vi "Get Magnet Field.vi"(6 "Axis":T1, 8 "error in (no error)":errorcluster, 11 "instrument.PPMS2 in":refnum<class "instrument.PPMS2.lvclass">) -> (0 "error out":errorcluster, 1 "Status":variant, 2 "B Field (T)":dbl, 3 "instrument.PPMS2 out":refnum<class "instrument.PPMS2.lvclass">, 4 "Finished?":bool)   [LabVIEW 2016, in "instrument.PPMS2.lvclass"]
uses:
  instrument.PPMS2.lvclass
  <userlib>/LevyLab/Levylab Instruments/Instrument Types/Cryostat/Typedefs/Magnet Axis--Enum.ctl
  Typedefs/PPMS2.Magnet Status--cluster.ctl
  Typedefs/PPMS2.Commands-enum.ctl
  <userlib>/LevyLab/Levylab Instruments/Instrument Types/Cryostat/Instrument.Cryostat.lvclass
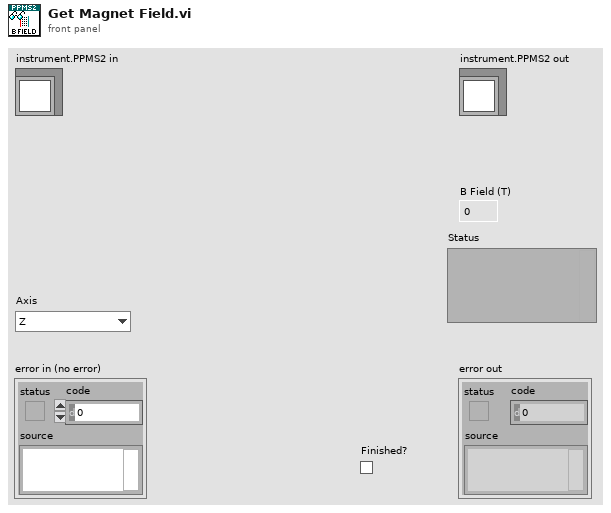
[diagram p1: front panel]
types:
  T1 = typedef "Instrument.Cryostat.lvclass/Magnet Axis--Enum.ctl" = enum16{"Z", "X", "Y"}
  T2 = typedef "instrument.PPMS2.lvclass/PPMS2.Commands-enum.ctl" = enum16{"Get Magnet Field", "Get Helium Level", "Get Temperature", "Get Angle", "Set Magnet Field", "Set Temperature", "Set Angle", "getAll"}
  T3 = typedef "instrument.PPMS2.lvclass/PPMS2.Magnet Status--cluster.ctl" = cluster{"Field (Oe)":dbl, "Magnet Status":string}
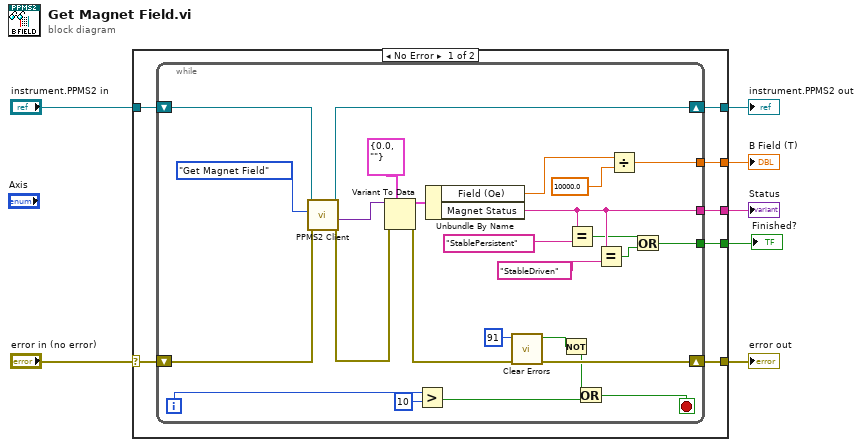
[diagram p0: block diagram]
diagram:
  n1 = case shown="No Error" "error in (no error)" {
    selector: "error in (no error)" -> [w9 w41]
    tunnel: [w10 w41] -> w7
    tunnel: [w14 w42] -> w6
    tunnel: "instrument.PPMS2 in" -> [w13 w42]
    tunnel: [w12 _] -> w4
    tunnel: [w11 _] -> w3
    tunnel: [w8 _] -> w1
    frame No Error {
      n2 = while {
        tunnel: [w25] -> w12
        tunnel: [w34] -> w11
        shift-right: [w29] -> w10
        shift-left: w9 -> [w39]
        shift-right: [w38] -> w14
        shift-left: w13 -> [w37]
        tunnel: [w21] -> w8
        i -> [w16]
        stop <- w15 stop-if-true
        n3 = call "PPMS2 Client.vi"("error in (no error)"=w39, "Command"=PPMS2.Commands-enum."Get Magnet Field" ("Enum"), "instrument.PPMS2 in"=w37) -> ("error out"=w30:errorcluster, "Data out"=w31:variant, "instrument.PPMS2 out"=w38:refnum<class "instrument.PPMS2.lvclass">)  [unwired: 5 in, 1 out]
        n4 = Variant To Data(error in=w30, type=T3 {"Field (Oe)"=0.0, "Magnet Status"=""} ("cluster"), Variant=w31) -> (data=w32:T3, error out=w40:errorcluster)
        n5 = Greater?(x=w16, y=10) -> (0:w19:bool)
        n6 = Unbundle By Name(w32) -> ("Field (Oe)"=w35:dbl, "Magnet Status"=w25:string)
        n7 = call <vilib>:"Clear Errors.vi"("error in (no error)"=w40, "specific error code to clear (0: all)"=91) -> ("error out"=w29:errorcluster, "specific error cleared?"=w17:bool)  [unwired: 4 in]
        n8 = Not(x=w17) -> (.not. x?=w18:bool)
        n9 = Equal?(x=w25, y="StablePersistent") -> (x = y?=w23:bool)
        n10 = Or(x=w18, y=w19) -> (x .or. y?=w15:bool)
        n11 = Equal?(x=w25, y="StableDriven") -> (x = y?=w22:bool)
        n12 = Divide(x=w35, y=10000.0) -> (x/y=w34:dbl)
        n13 = Or(x=w23, y=w22) -> (x .or. y?=w21:bool)
      }
    }
    frame Error {
    }
  }
  "error out" <- w7
  "instrument.PPMS2 out" <- w6
  "B Field (T)" <- w3
  "Status" <- w4
  "Finished?" <- w1
